vi "FromToMachineToArray.vi"(10 "string":string) -> (2 "array":string[](array[string]))   [LabVIEW 2012]
panel:
  out "after substring 2":string
  out "number":i32
  out "after substring":string
  out "before substring":string
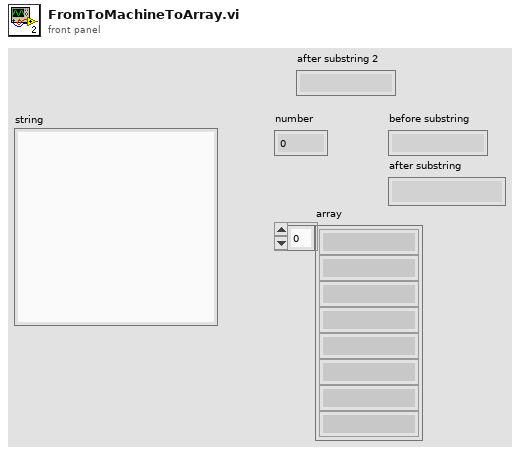
[diagram p1: front panel]
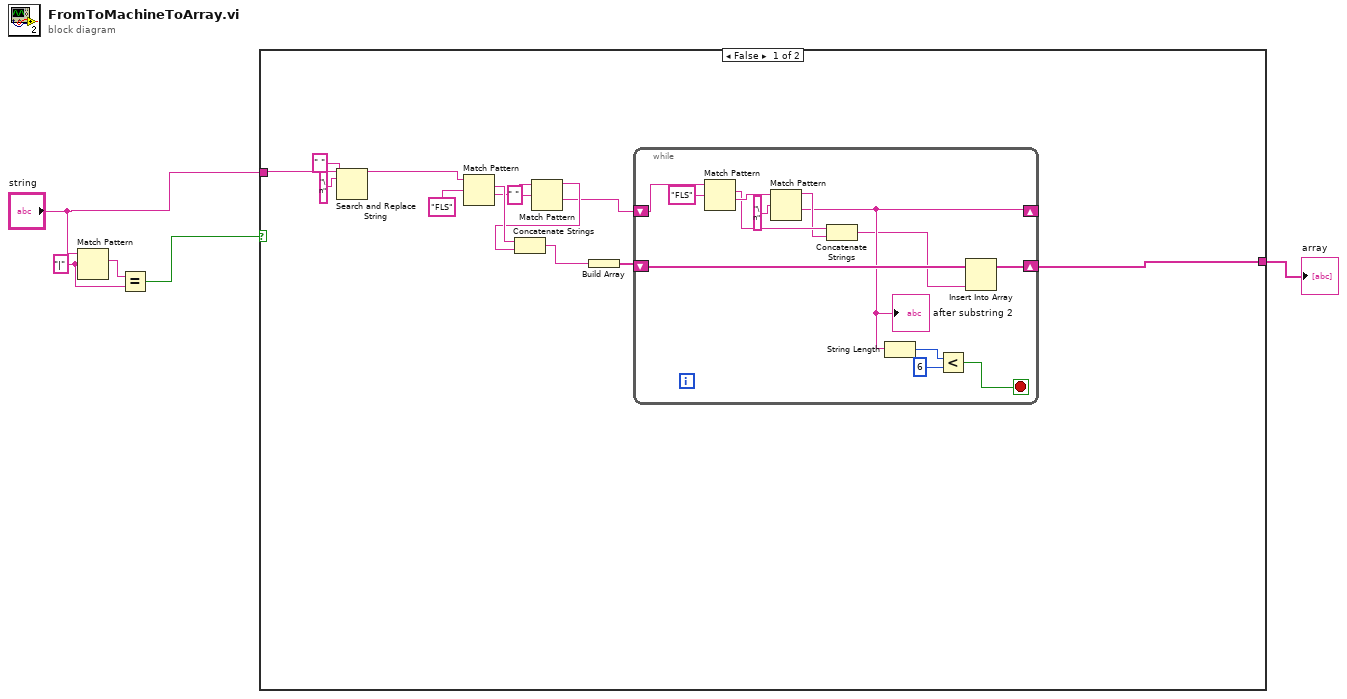
[diagram p0: block diagram]
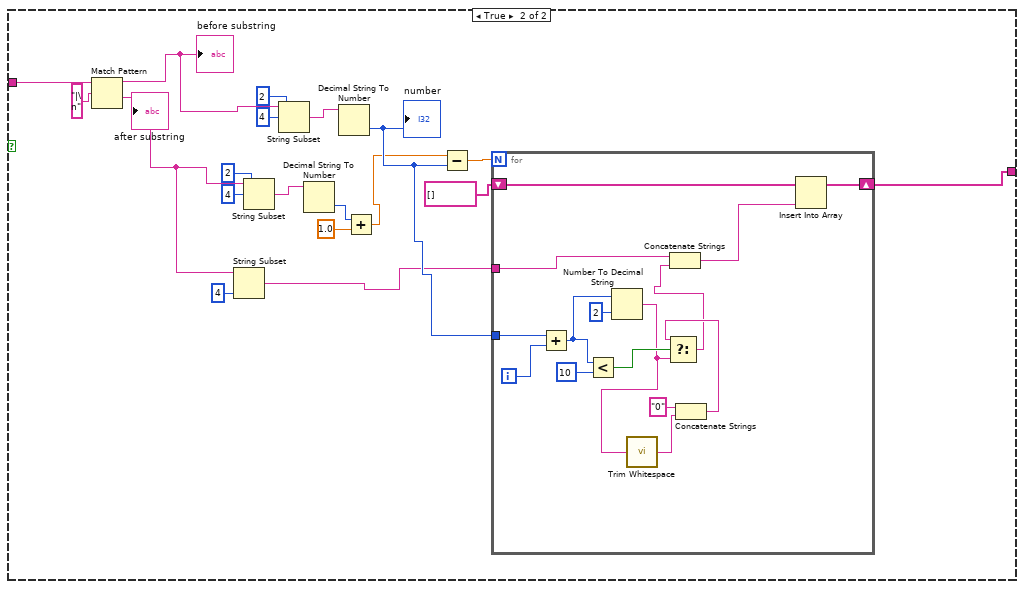
[diagram p2: hidden frame]
diagram:
  w3 = "|" ("regular expression")
  n1 = Match Pattern(string="string", regular expression=w3) -> (match substring=w4:string)  [unwired: 1 in, 3 out]
  n2 = Equal?(x=w4, y=w3) -> (x = y?=w2:bool)
  n3 = case shown="False" w2 {
    tunnel: "string" -> [w9 w50]
    tunnel: [w10 w32] -> w1
    frame False {
      n4 = Search and Replace String(input string=w9, search string="\n", replace string=" " ("replace string (\"\")")) -> (result string=w8:string)  [unwired: 5 in, 3 out]
      n5 = Match Pattern(string=w8, regular expression="FLS" ("replace string (\"\")")) -> (match substring=w17:string, after substring=w16:string)  [unwired: 1 in, 2 out]
      n6 = Match Pattern(string=w16, regular expression=" ") -> (before substring=w14:string, after substring=w11:string)  [unwired: 1 in, 2 out]
      n7 = Concatenate Strings(w17, w14) -> (w13:string)
      n8 = Build Array(w13) -> (w12:string[])
      n9 = while {
        shift-right: [w31] -> w10
        shift-left: w12 -> [w30]
        shift-right: [w23] -> _
        shift-left: w11 -> [w24]
        stop <- w20 stop-if-true
        n10 = Match Pattern(string=w24, regular expression="FLS") -> (match substring=w26:string, after substring=w28:string)  [unwired: 1 in, 2 out]
        n11 = Match Pattern(string=w28, regular expression="\n") -> (before substring=w25:string, after substring=w23:string)  [unwired: 1 in, 2 out]
        "after substring 2" <- w23
        n12 = Concatenate Strings(w26, w25) -> (w19:string)
        n13 = String Length(string=w23) -> (length=w22:i32)
        n14 = Less?(x=w22, y=6) -> (x < y?=w20:bool)
        n15 = Insert Into Array(array=w30, new element=w19) -> (w31:string[])  [unwired: 1 in]
      }
    }
    frame True {
      n16 = Match Pattern(string=w50, regular expression="|\n") -> (before substring=w48:string, after substring=w36:string)  [unwired: 1 in, 2 out]
      "before substring" <- w48
      "after substring" <- w36
      n17 = String Subset(string=w36, length (rest)=4 ("length (rest)")) -> (substring=w34:string)  [unwired: 1 in]
      n18 = String Subset(string=w36, offset (0)=4, length (rest)=2 ("length (rest)")) -> (substring=w42:string)
      n19 = String Subset(string=w48, offset (0)=4, length (rest)=2 ("length (rest)")) -> (substring=w45:string)
      n20 = Decimal String To Number(string=w42) -> (number=w38:i32)  [unwired: 2 in, 1 out]
      n21 = Decimal String To Number(string=w45) -> (number=w40:i32)  [unwired: 2 in, 1 out]
      "number" <- w40
      n22 = Add(x=w38, y=1.0) -> (x+y=w37:dbl)
      n23 = Subtract(x=w37, y=w40) -> (x-y=w41:dbl)
      n24 = for {
        N: w41 -> [_]
        tunnel: w40 -> [w65]
        tunnel: w34 -> [w63]
        shift-right: [w52] -> w32
        shift-left: string[] [] ("array") -> [w51]
        i -> [w64]
        n25 = Add(x=w65, y=w64) -> (x+y=w61:i32)
        n26 = Less?(x=w61, y=10) -> (x < y?=w59:bool)
        n27 = Number To Decimal String(number=w61, width (-)=i16 2) -> (decimal integer string=w57:string)
        n28 = call <vilib>:"Trim Whitespace.vi"("string"=w57) -> ("trimmed string"=w56:string)  [unwired: 1 in]
        n29 = Concatenate Strings("0" ("string"), w56) -> (w55:string)
        n30 = Select(t=w55, s=w59, f=w57) -> (s? t:f=w54:string)
        n31 = Concatenate Strings(w63, w54) -> (w53:string)
        n32 = Insert Into Array(array=w51, new element=w53) -> (w52:string[])  [unwired: 1 in]
      }
    }
  }
  "array" <- w1
